vi "Flatten.vi"(6 "Persistence in":refnum<class "IPersist.lvclass">, 7 "Linked List Ref":refnum<data-value>, 8 "error in (no error)":errorcluster, 9 "Indent":i32, 10 "Active Unique ID":string, 11 "Subroutine in":refnum<class "Subroutine.lvclass">) -> (0 "error out":errorcluster, 2 "Active Unique ID out":string, 3 "Flattened Test Executive":string[](array[string]), 4 "Persistence out":refnum<class "IPersist.lvclass">, 5 "Linked List Ref out":refnum<data-value>)   [LabVIEW 2020, in "Test Executive.lvlib" / "Subroutine.lvclass"]
uses:
  <vilib>/gpm_packages/@cs/test-executive/Source/Test Executive/Subroutine/Subroutine.lvclass
  <vilib>/gpm_packages/@cs/linked-list/Source/Linked List/ILinkedList/ILinked List.lvclass
  <vilib>/gpm_packages/@cs/persistence/source/IPersist/IPersist.lvclass
  <vilib>/gpm_packages/@cs/linked-list/Source/Linked List/Linked List Ref/Linked List Ref.lvclass
  <vilib>/gpm_packages/@cs/linked-list/Source/String Manipulation/String Manipulation.lvlib
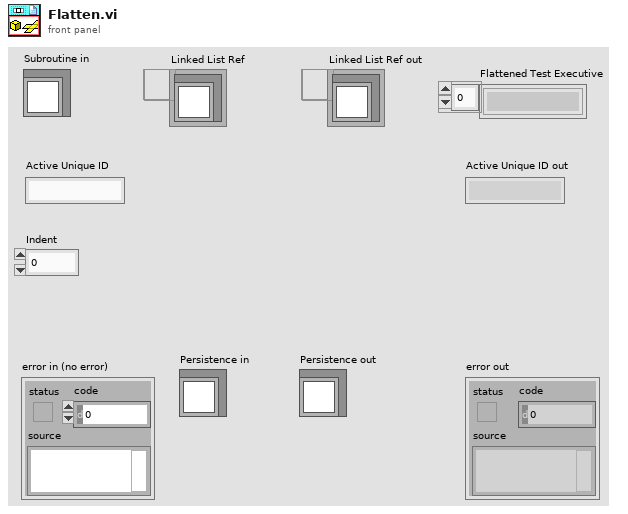
[diagram p1: front panel]
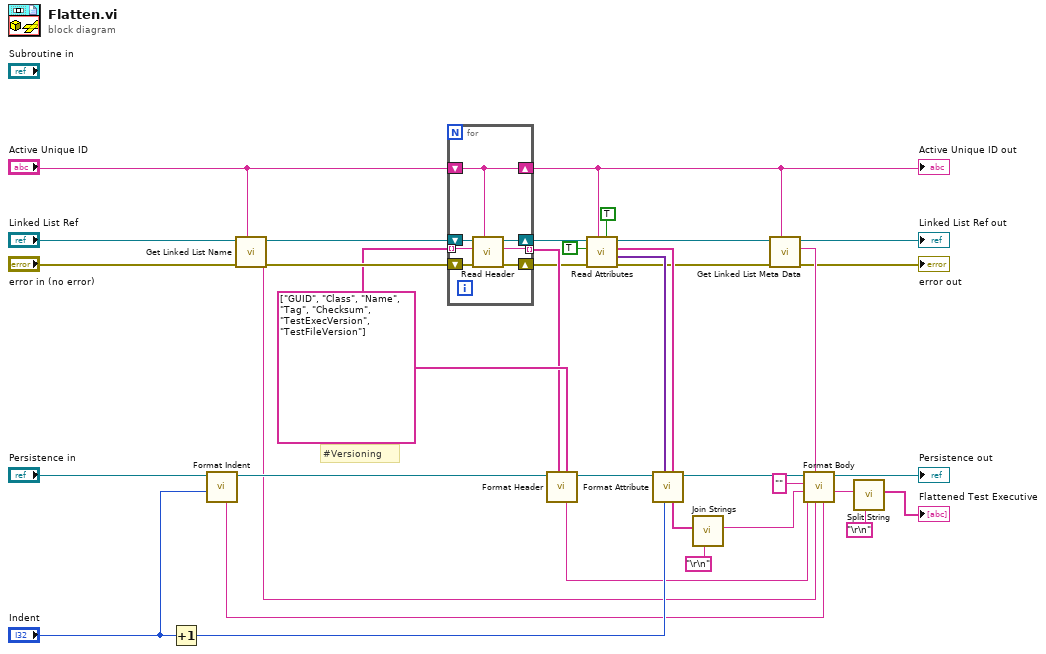
[diagram p0: block diagram]
diagram:
  w33 = string[] ["GUID", "Class", "Name", "Tag", "Checksum", "TestExecVersion", "TestFileVersion"] ("Header Names")
  # "#Versioning"
  n1 = Increment(x="Indent") -> (x+1=w23:i32)
  n2 = call-dynamic "Format Indent.vi"("Indent"="Indent", "IPersist in"="Persistence in") -> ("IPersist out"=w34:refnum<class "IPersist.lvclass">, "Indent XML"=w15:string)  [unwired: 7 in, 1 out]
  n3 = call <vilib>:"Get Linked List Name.vi"("Linked List ID"="Active Unique ID", "error in (no error)"="error in (no error)", "Linked List Ref"="Linked List Ref") -> ("error out"=w35:errorcluster, "Linked List Name"=w16:string, "Linked List Ref out"=w36:refnum<data-value>)  [unwired: 5 in, 1 out]
  n4 = for {
    tunnel: w33 -> [w41] mode=indexing
    shift-right: [w42] -> w26
    shift-left: w36 -> [w43]
    tunnel: [w40] -> w32 mode=indexing
    shift-right: [w39] -> w2
    shift-left: "Active Unique ID" -> [w39]
    shift-right: [w37] -> w25
    shift-left: w35 -> [w38]
    n5 = call <vilib>:"Read Header.vi"("Linked List ID"=w39, "error in (no error)"=w38, "Header Name"=w41, "Linked List Ref"=w43) -> ("error out"=w37:errorcluster, "Header Value"=w40:string, "Linked List Ref out"=w42:refnum<data-value>)  [unwired: 4 in, 1 out]
  }
  "Active Unique ID out" <- w2
  n6 = call-dynamic "Format Header.vi"("Name"=w33, "Value"=w32, "IPersist in"=w34) -> ("IPersist out"=w24:refnum<class "IPersist.lvclass">, "Header"=w17:string)  [unwired: 7 in]
  n7 = call <vilib>:"Read Attributes.vi"("Flatten Pointer?"=TRUE, "Linked List ID"=w2, "error in (no error)"=w25, "Include Private?"=TRUE, "Linked List Ref"=w26) -> ("error out"=w13:errorcluster, "Attributes"=w30:variant[], "Attribute Names out"=w29:string[], "Linked List Ref out"=w14:refnum<data-value>)  [unwired: 1 in, 2 out]
  n8 = call-dynamic "Format Attribute.vi"("Attribute Names"=w29, "Indent"=w23, "Attribute Values"=w30, "IPersist in"=w24) -> ("IPersist out"=w19:refnum<class "IPersist.lvclass">, "Attr Strings"=w27:string[])  [unwired: 6 in]
  n9 = call <vilib>:"Join Strings.vi"("Separator (,)"="\r\n", "Strings In"=w27) -> ("String"=w18:string)  [unwired: 9 in]
  n10 = call <vilib>:"Get Linked List Meta Data.vi"("Linked List ID"=w2, "error in (no error)"=w13, "Linked List Ref"=w14) -> ("error out"=→"error out":errorcluster, "Meta Data"=w22:string, "Linked List Ref out"=→"Linked List Ref out":refnum<data-value>)  [unwired: 5 in, 1 out]
  n11 = call-dynamic "Format Body.vi"("Indent"=w15, "Name"=w16, "Meta Data"=w22, "Header"=w17, "Attributes"=w18, "Body"="", "IPersist in"=w19) -> ("String out"=w20:string, "IPersist out"=→"Persistence out":refnum<class "IPersist.lvclass">)  [unwired: 3 in]
  n12 = call <vilib>:"Split String.vi"("Split Pattern"="\r\n", "Input String"=w20) -> ("Split String"=→"Flattened Test Executive":string[])  [unwired: 9 in]
